vi "PWM12.vi"(11 "Percent Power":dbl format="%#_13g") -> ()   [LabVIEW 2019]
panel:
  out "error out 2":errorcluster
  out "error out":errorcluster
  in  "error in (no error) 2":errorcluster
  in  "error in (no error)":errorcluster
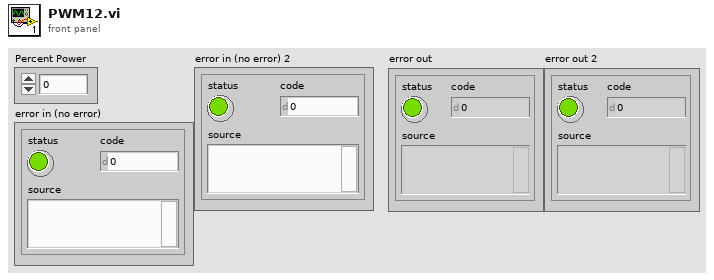
[diagram p1: front panel]
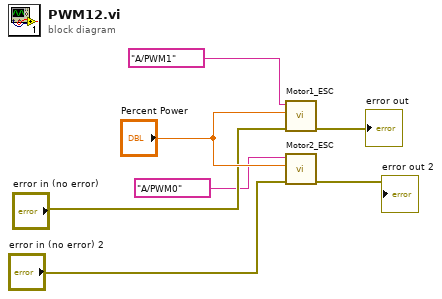
[diagram p0: block diagram]
diagram:
  n1 = call "Motor1_ESC.vi"("error in (no error)"="error in (no error)", "Percent Power"="Percent Power", "Channel Name"=tag "A/PWM1") -> ("error out"=→"error out":errorcluster)  [unwired: 8 in]
  n2 = call "Motor2_ESC.vi"("error in (no error)"="error in (no error) 2", "Percent Power"="Percent Power", "Channel Name"=tag "A/PWM0") -> ("error out"=→"error out 2":errorcluster)  [unwired: 8 in]
